vi "Swerve Motor Setup.vi"() -> (2 "Finished":bool=TRUE)   [LabVIEW 2016]
uses:
  <vilib>/Rock Robotics/WPI/ThirdParty/CanMotor/TalonSRX/WPI_CANTalonSRX_APIControlMode.ctl
  <vilib>/Rock Robotics/WPI/ThirdParty/CanMotor/TalonSRX/WPI_CANTalonSRX_BrakeOverride.ctl
  <vilib>/Rock Robotics/WPI/SafetyOutput/WPI_SafetyOutputConfigMenu.ctl
  <vilib>/Rock Robotics/WPI/ThirdParty/CanMotor/TalonSRX/WPI_CANTalonSRX_APIFeedbackSelect.ctl
  Robot Global Data.vi
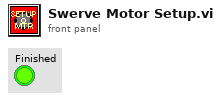
[diagram p1: front panel]
types:
  T1 = enum16{"Can ID", "P", "I", "D", "F", "IZone", "RampSpeed", "Fwd speed Limit", "Rev Speed Limit", "InvertDrive"}
  T2 = typedef "WPI_CANTalonSRX_BrakeOverride.ctl" = enum8{"No Override", "Override to Coast", "Override to Brake"}
  T3 = typedef "WPI_CANTalonSRX_APIControlMode.ctl" = enum8{"Percent VBus", "Speed", "Position", "Slave", "Unchanged / Invalid", "Voltage Compensation", "Current", "Motion Profile", "Motion Magic"}
  T4 = enum16{"FL Drive Wheel", "FR Drive Wheel", "RL Drive Wheel", "RR Drive Wheel", "FL Steer Wheel", "FR Steer Wheel", "RL Steer Wheel", "RR Steer Wheel"}
  T5 = typedef "WPI_SafetyOutputConfigMenu.ctl" = enum16{"Enable", "Disable"}
  T6 = typedef "WPI_CANTalonSRX_APIFeedbackSelect.ctl" = enum16{"Digital Quadrature Encoder", "Analog Potentiometer", "Analog Encoder", "Count on Quad-A (Rising-Edge)", "Count on Quad-A (Falling-Edge)", "CTR Magnetic Enc (Absolute)", "CTR Magnetic Enc (Relative)", "Pulse Width"}
  T7 = typedef "WPI_MotorControlDeviceRef.ctl" = cluster{"DeviceStatus":errorcluster, "Type":T8, "PWM":cluster{"PWM Channel":T9, "DeadBand":T10}, "CAN":cluster{"Device Number":u8, "SetOutput VI Ref":variant, "GetOutput VI Ref":variant, "Enable VI Ref":variant, "Disable VI Ref":variant, "Data":variant}, "Invert":bool}
  T8 = typedef "WPI_MotorControlType.ctl" = enum16{"PWM", "CAN"}
  T9 = typedef "FPGA_DIOPWMChannel.ctl" = enum8{"PWM 0", "PWM 1", "PWM 2", "PWM 3", "PWM 4", "PWM 5", "PWM 6", "PWM 7", "PWM 8", "PWM 9", "PWM MXP 0", "PWM MXP 1", "PWM MXP 2", "PWM MXP 3", "PWM MXP 4", "PWM MXP 5", "PWM MXP 6", "PWM MXP 7", "PWM MXP 8", "PWM MXP 9", "Invalid"}
  T10 = typedef "WPI_PWMDeadband.ctl" = cluster{"Name":string, "maxPositivePwm":i32, "minPositivePwm":i32, "centerPwm":i32, "maxNegativePwm":i32, "minNegativePwm":i32, "angularRange":u16}
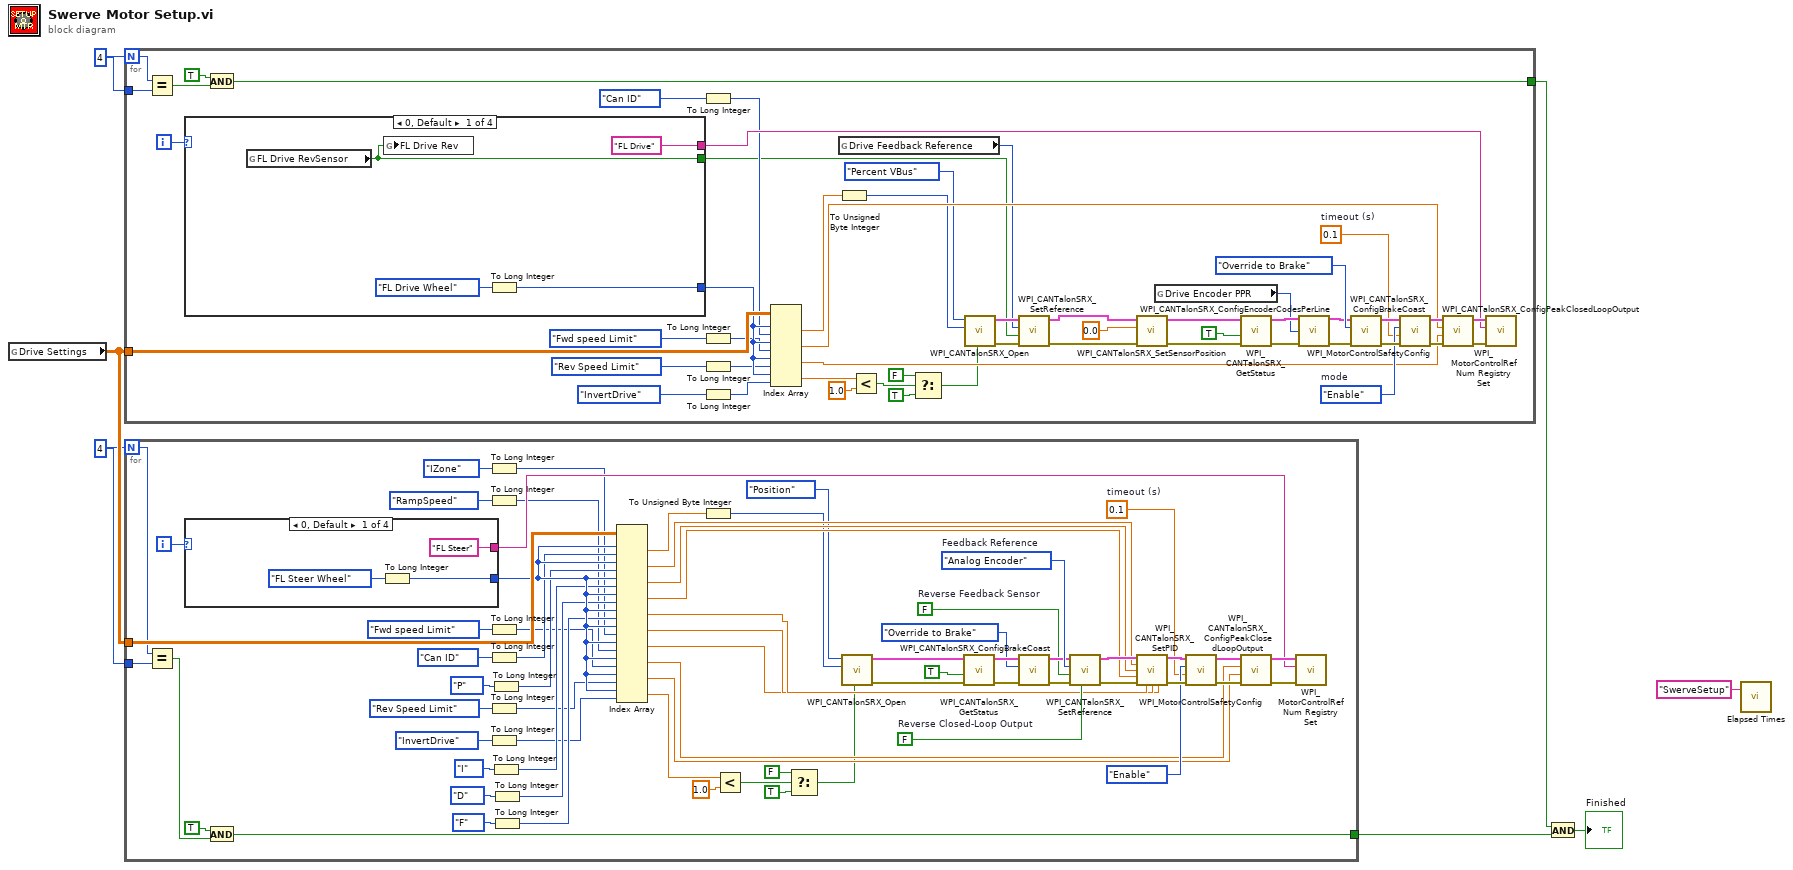
[diagram p0: block diagram]
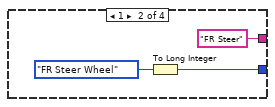
[diagram p2: hidden frame]
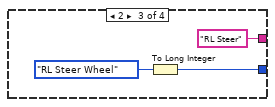
[diagram p3: hidden frame]
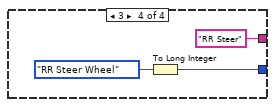
[diagram p4: hidden frame]
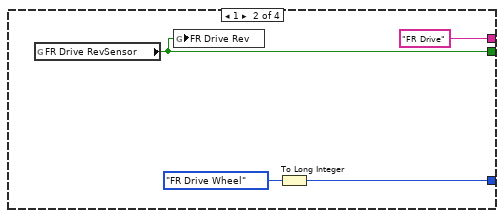
[diagram p5: hidden frame]
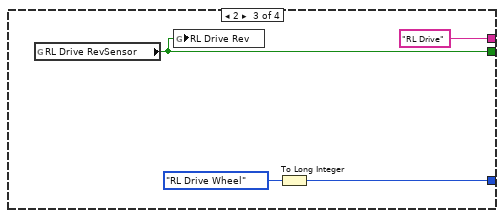
[diagram p6: hidden frame]
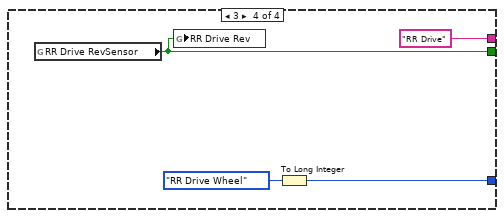
[diagram p7: hidden frame]
diagram:
  w3 = 4
  w2 = 4
  n1 = global read "Robot Global Data.vi" "Drive Settings"() -> (w7:dbl[][])
  n2 = for {
    N: w2 -> [w40]
    tunnel: w7 -> [w45]
    tunnel: [w39] -> w6
    tunnel: w2 -> [w41]
    i -> [w59]
    w55 = WPI_SafetyOutputConfigMenu."Enable"  # mode
    w54 = 0.1  # timeout (s)
    n3 = Equal?(x=w40, y=w41) -> (x = y?=w42:bool)
    n4 = case shown="0, Default" w59 {
      tunnel: [w63 w66 w70 w74] -> w36
      tunnel: ["FL Drive" ("refnum name") "FR Drive" ("refnum name") "RL Drive" ("refnum name") "RR Drive" ("refnum name")] -> w44
      tunnel: [w60 w64 w68 w72] -> w14
      frame 0, Default {
        n5 = global read "Robot Global Data.vi" "FL Drive RevSensor"() -> (w60:bool)
        n6 = global write "Robot Global Data.vi" "FL Drive Rev"(w60) -> ()
        n7 = To Long Integer(number=T4."FL Drive Wheel" ("Swerve Drive Param")) -> (32bit integer=w63:i32)
      }
      frame 1 {
        n8 = global read "Robot Global Data.vi" "FR Drive RevSensor"() -> (w64:bool)
        n9 = global write "Robot Global Data.vi" "FR Drive Rev"(w64) -> ()
        n10 = To Long Integer(number=T4."FR Drive Wheel" ("Swerve Drive Param")) -> (32bit integer=w66:i32)
      }
      frame 2 {
        n11 = global read "Robot Global Data.vi" "RL Drive RevSensor"() -> (w68:bool)
        n12 = global write "Robot Global Data.vi" "RL Drive Rev"(w68) -> ()
        n13 = To Long Integer(number=T4."RL Drive Wheel" ("Swerve Drive Param")) -> (32bit integer=w70:i32)
      }
      frame 3 {
        n14 = global read "Robot Global Data.vi" "RR Drive RevSensor"() -> (w72:bool)
        n15 = global write "Robot Global Data.vi" "RR Drive Rev"(w72) -> ()
        n16 = To Long Integer(number=T4."RR Drive Wheel" ("Swerve Drive Param")) -> (32bit integer=w74:i32)
      }
    }
    n17 = And(x=TRUE, y=w42) -> (x .and. y?=w39:bool)
    n18 = To Long Integer(number=T1."Can ID" ("Enum")) -> (32bit integer=w34:i32)
    n19 = To Long Integer(number=T1."Fwd speed Limit" ("Enum")) -> (32bit integer=w30:i32)
    n20 = To Long Integer(number=T1."Rev Speed Limit" ("Enum")) -> (32bit integer=w33:i32)
    n21 = To Long Integer(number=T1."InvertDrive" ("Enum")) -> (32bit integer=w32:i32)
    n22 = Index Array(array=w45, index (row) #1=w36, index (col) #1=w34, index (row) #2=w36, index (col) #2=w30, index (row) #3=w36, index (col) #3=w33, index (row) #4=w36, index (col) #4=w32) -> (element #1=w48:dbl, element #2=w47:dbl, element #3=w46:dbl, element #4=w28:dbl)
    n23 = global read "Robot Global Data.vi" "Drive Feedback Reference"() -> (w13:T6)
    n24 = To Unsigned Byte Integer(number=w48) -> (unsigned 8bit integer=w23:u8)
    n25 = Less?(x=w28, y=1.0) -> (x < y?=w27:bool)
    n26 = Select(t=FALSE, s=w27, f=TRUE) -> (s? t:f=w22:bool)
    n27 = call <vilib>:"WPI_CANTalonSRX_Open.vi"("Invert"=w22, "Device Number"=w23, "Control Mode"=WPI_CANTalonSRX_APIControlMode."Percent VBus") -> ("error out"=w15:errorcluster, "CAN Talon SRX Ref"=w16:T7)  [unwired: 7 in]
    n28 = call <vilib>:"WPI_CANTalonSRX_SetReference.vi"("error in (no error)"=w15, "Reverse Feedback Sensor"=w14, "Feedback Reference"=w13, "CAN Talon SRX Ref"=w16) -> ("error out"=w12:errorcluster, "CAN Talon SRX Ref"=w11:T7)  [unwired: 6 in]
    n29 = call <vilib>:"WPI_CANTalonSRX_SetSensorPosition.vi"("error in (no error)"=w12, "New Sensor Position"=0.0, "CAN Talon SRX Ref"=w11) -> ("error out"=w9:errorcluster, "CAN Talon SRX Ref"=w10:T7)  [unwired: 7 in]
    n30 = global read "Robot Global Data.vi" "Drive Encoder PPR"() -> (w17:u32)
    n31 = call <vilib>:"WPI_CANTalonSRX_GetStatus.vi"("error in (no error)"=w9, "Clear Sticky Faults"=TRUE, "CAN Talon SRX Ref"=w10) -> ("error out"=w21:errorcluster, "CAN Talon SRX Ref"=w20:T7)  [unwired: 6 in, 1 out]
    n32 = call <vilib>:"WPI_CANTalonSRX_ConfigEncoderCodesPerLine.vi"("CAN Talon SRX Ref"=w20, "Number Encoder Lines\n(Counts Per Rotation)"=w17, "error in (no error)"=w21) -> ("CAN Talon SRX Ref"=w19:T7, "error out"=w18:errorcluster)  [unwired: 11 in]
    n33 = call <vilib>:"WPI_CANTalonSRX_ConfigBrakeCoast.vi"("error in (no error)"=w18, "Brake / Coast Mode"=WPI_CANTalonSRX_BrakeOverride."Override to Brake", "CAN Talon SRX Ref"=w19) -> ("error out"=w56:errorcluster, "CAN Talon SRX Ref"=w57:T7)  [unwired: 7 in]
    n34 = call <vilib>:"WPI_MotorControlSafetyConfig.vi"("error in (no error)"=w56, "timeout (s)"=w54, "mode"=w55, "MotorControlDevRef"=w57) -> ("error out"=w51:errorcluster, "MotorControlDevRef"=w52:T7)  [unwired: 6 in]
    n35 = call <vilib>:"WPI_CANTalonSRX_ConfigPeakClosedLoopOutput.vi"("error in (no error)"=w51, "Reverse Peak Output"=w46, "Forward Peak Output"=w47, "CAN Talon SRX Ref"=w52) -> ("error out"=w49:errorcluster, "CAN Talon SRX Ref"=w50:T7)  [unwired: 6 in]
    n36 = call <vilib>:"WPI_MotorControlRefNum Registry Set.vi"("error in (no error)"=w49, "refnum name"=w44, "MotorControlDevRef"=w50) -> ()  [unwired: 7 in, 2 out]
  }
  n37 = for {
    N: w3 -> [w111]
    tunnel: w7 -> [w114]
    tunnel: [w107] -> w5
    tunnel: w3 -> [w110]
    i -> [w113]
    w128 = 0.1  # timeout (s)
    w134 = FALSE  # Reverse Closed-Loop Output
    w135 = FALSE  # Reverse Feedback Sensor
    w138 = WPI_CANTalonSRX_APIFeedbackSelect."Analog Encoder"  # Feedback Reference
    n38 = Equal?(x=w111, y=w110) -> (x = y?=w108:bool)
    n39 = case shown="0, Default" w113 {
      tunnel: [w145 w148 w150 w152] -> w106
      tunnel: ["FL Steer" ("refnum name") "FR Steer" ("refnum name") "RL Steer" ("refnum name") "RR Steer" ("refnum name")] -> w112
      frame 0, Default {
        n40 = To Long Integer(number=T4."FL Steer Wheel" ("Swerve Drive Param")) -> (32bit integer=w145:i32)
      }
      frame 1 {
        n41 = To Long Integer(number=T4."FR Steer Wheel" ("Swerve Drive Param")) -> (32bit integer=w148:i32)
      }
      frame 2 {
        n42 = To Long Integer(number=T4."RL Steer Wheel" ("Swerve Drive Param")) -> (32bit integer=w150:i32)
      }
      frame 3 {
        n43 = To Long Integer(number=T4."RR Steer Wheel" ("Swerve Drive Param")) -> (32bit integer=w152:i32)
      }
    }
    n44 = And(x=TRUE, y=w108) -> (x .and. y?=w107:bool)
    n45 = To Long Integer(number=T1."IZone" ("Enum")) -> (32bit integer=w90:i32)
    n46 = To Long Integer(number=T1."RampSpeed" ("Enum")) -> (32bit integer=w86:i32)
    n47 = To Long Integer(number=T1."Fwd speed Limit" ("Enum")) -> (32bit integer=w89:i32)
    n48 = To Long Integer(number=T1."Can ID" ("Enum")) -> (32bit integer=w95:i32)
    n49 = To Long Integer(number=T1."Rev Speed Limit" ("Enum")) -> (32bit integer=w88:i32)
    n50 = To Long Integer(number=T1."InvertDrive" ("Enum")) -> (32bit integer=w87:i32)
    n51 = To Long Integer(number=T1."P" ("Enum")) -> (32bit integer=w94:i32)
    n52 = To Long Integer(number=T1."I" ("Enum")) -> (32bit integer=w93:i32)
    n53 = To Long Integer(number=T1."D" ("Enum")) -> (32bit integer=w92:i32)
    n54 = To Long Integer(number=T1."F" ("Enum")) -> (32bit integer=w91:i32)
    n55 = Index Array(array=w114, index (row) #1=w106, index (col) #1=w95, index (row) #2=w106, index (col) #2=w94, index (row) #3=w106, index (col) #3=w93, index (row) #4=w106, index (col) #4=w92, index (row) #5=w106, index (col) #5=w91, index (row) #6=w106, index (col) #6=w90, index (row) #7=w106, index (col) #7=w86, index (row) #8=w106, index (col) #8=w89, index (row) #9=w106, index (col) #9=w88, index (row) #10=w106, index (col) #10=w87) -> (element #1=w123:dbl, element #2=w122:dbl, element #3=w121:dbl, element #4=w120:dbl, element #5=w119:dbl, element #6=w118:dbl, element #7=w117:dbl, element #8=w116:dbl, element #9=w115:dbl, element #10=w81:dbl)
    n56 = To Unsigned Byte Integer(number=w123) -> (unsigned 8bit integer=w79:u8)
    n57 = Less?(x=w81, y=1.0) -> (x < y?=w84:bool)
    n58 = Select(t=FALSE, s=w84, f=TRUE) -> (s? t:f=w78:bool)
    n59 = call <vilib>:"WPI_CANTalonSRX_Open.vi"("Invert"=w78, "Device Number"=w79, "Control Mode"=WPI_CANTalonSRX_APIControlMode."Position") -> ("error out"=w77:errorcluster, "CAN Talon SRX Ref"=w76:T7)  [unwired: 7 in]
    n60 = call <vilib>:"WPI_CANTalonSRX_GetStatus.vi"("error in (no error)"=w77, "Clear Sticky Faults"=TRUE, "CAN Talon SRX Ref"=w76) -> ("error out"=w141:errorcluster, "CAN Talon SRX Ref"=w140:T7)  [unwired: 6 in, 1 out]
    n61 = call <vilib>:"WPI_CANTalonSRX_ConfigBrakeCoast.vi"("error in (no error)"=w141, "Brake / Coast Mode"=WPI_CANTalonSRX_BrakeOverride."Override to Brake", "CAN Talon SRX Ref"=w140) -> ("error out"=w136:errorcluster, "CAN Talon SRX Ref"=w137:T7)  [unwired: 7 in]
    n62 = call <vilib>:"WPI_CANTalonSRX_SetReference.vi"("Reverse Closed-Loop Output"=w134, "error in (no error)"=w136, "Reverse Feedback Sensor"=w135, "Feedback Reference"=w138, "CAN Talon SRX Ref"=w137) -> ("error out"=w132:errorcluster, "CAN Talon SRX Ref"=w133:T7)  [unwired: 5 in]
    n63 = call <vilib>:"WPI_CANTalonSRX_SetPID.vi"("CAN Talon SRX Ref"=w133, "P"=w122, "I"=w121, "D"=w120, "error in (no error)"=w132, "F"=w119, "I Zone"=w118, "Ramp Rate"=w117) -> ("CAN Talon SRX Ref"=w130:T7, "error out"=w131:errorcluster)  [unwired: 6 in]
    n64 = call <vilib>:"WPI_MotorControlSafetyConfig.vi"("error in (no error)"=w131, "timeout (s)"=w128, "mode"=WPI_SafetyOutputConfigMenu."Enable", "MotorControlDevRef"=w130) -> ("error out"=w127:errorcluster, "MotorControlDevRef"=w126:T7)  [unwired: 6 in]
    n65 = call <vilib>:"WPI_CANTalonSRX_ConfigPeakClosedLoopOutput.vi"("error in (no error)"=w127, "Reverse Peak Output"=w115, "Forward Peak Output"=w116, "CAN Talon SRX Ref"=w126) -> ("error out"=w124:errorcluster, "CAN Talon SRX Ref"=w125:T7)  [unwired: 6 in]
    n66 = call <vilib>:"WPI_MotorControlRefNum Registry Set.vi"("error in (no error)"=w124, "refnum name"=w112, "MotorControlDevRef"=w125) -> ()  [unwired: 7 in, 2 out]
  }
  n67 = And(x=w6, y=w5) -> (x .and. y?=→"Finished":bool)
  n68 = call "Elapsed Times.vi"("Call Name"="SwerveSetup") -> ()  [unwired: 2 in, 1 out]
